vi "Init.vi"() -> (3 "Setup Msg Strategy out":refnum<class "Setup Msg Strategy.lvclass">)   [LabVIEW 2021, in "jettl Msg Setup.lvlib" / "Setup Msg Strategy.lvclass"]
uses:
  Setup Msg Strategy.lvclass
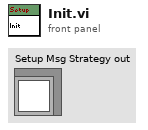
[diagram p1: front panel]
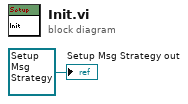
[diagram p0: block diagram]
diagram:
  "Setup Msg Strategy out" <- refnum<class "Setup Msg Strategy.lvclass"> refnum ("Setup Msg out")
